vi "Send MSG to Caller.vi"(8 "error in":errorcluster, 10 "Message":refnum<class "Message.lvclass">, 11 "Instr in":refnum<class "Instr Actor.lvclass">) -> (0 "error out":errorcluster, 3 "Instr out":refnum<class "Instr Actor.lvclass">)   [LabVIEW 2014, in "Instrument Library.lvlib" / "Instr Actor.lvclass"]
uses:
  Instr Actor.lvclass
  <vilib>/ActorFramework/Message/Message.lvclass
  <vilib>/ActorFramework/Actor/Actor.lvclass/Actor.ctl
  <vilib>/ActorFramework/Message Enqueuer/Message Enqueuer.lvclass/Message Enqueuer.ctl
  <vilib>/ActorFramework/Message Priority Queue/Priority Enqueue.vi
  <vilib>/ActorFramework/Actor/Actor.lvclass
  <vilib>/ActorFramework/Message Enqueuer/Message Enqueuer.lvclass
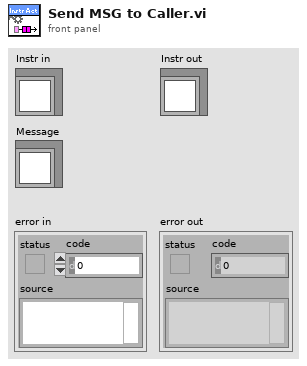
[diagram p1: front panel]
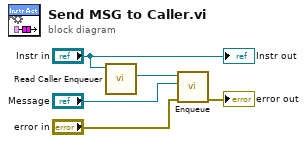
[diagram p0: block diagram]
diagram:
  n1 = call <vilib>:"Read Caller Enqueuer.vi"("Actor"="Instr in") -> ("Caller Enqueuer"=w4:refnum<class "Message Enqueuer.lvclass">)  [unwired: 10 in]
  n2 = call <vilib>:"Enqueue.vi"("error in (no error)"="error in", "Message"="Message", "Message Enqueuer in"=w4) -> ("error out"=→"error out":errorcluster)  [unwired: 7 in, 1 out]
  "Instr out" <- "Instr in"
